vi "IMAQdxCam-Fast-TIFF.vi"() -> ()   [LabVIEW 2011]
uses:
  <vilib>/vision/driver/IMAQdx.llb/IMAQdx Acquisition Mode.ctl
  <vilib>/vision/driver/IMAQdx.llb/IMAQdx Buffer Number Mode.ctl
  tiff/TiffModules/AddTiffPage_U8_text_res.vi
  tiff/TiffModules/AddTiffPage_I16_text_res.vi
  <vilib>/vision/driver/NI_Vision_Acquisition_Software.lvlib
  C:/Program Files/National Instruments/LabVIEW 2011/resource/objmgr/imaqdx.rc
  C:/Program Files/National Instruments/LabVIEW 2011/resource/objmgr/IMAQImage.rc
panel:
  in  "Exposure":dbl(slide)=2689.598785575046 scale=100.0..100000.0
  in  "IMAQdx-Session":string="cam0"
  in  "expected images":u32=1
  out "msperframe":u32(graph)
  out "measured":i32
  out "saved":i32
  out "Buffer Number Out":u32
  out "IFDoffset":u32
  out "Image Type":i32(ring) items=["8 bits", "16 bits", "Float", "Complex", "RGB", "HSL"]
  out "measuredloop":i32
  in  "tiff-file":path=path "C:/temp/test1.tif"
  out "error out":errorcluster
  # "init the cam in MAX first!"
  # "wait for trigger will be enabled\nacquire as fast as possible to RAM (IMAQs)\nno diplay, \nsave afterwards"
  # "usually µs"
  # "0..."
  # "fast 8bit 3920x1848 1000us\ntested 7x50 (36,3fps 27ms)"
  # "I16 and U8 tested!\nwill overwrite! no append"
  # "init an test the cam with NiMax first! Find Session name\ngo gain etc with other"
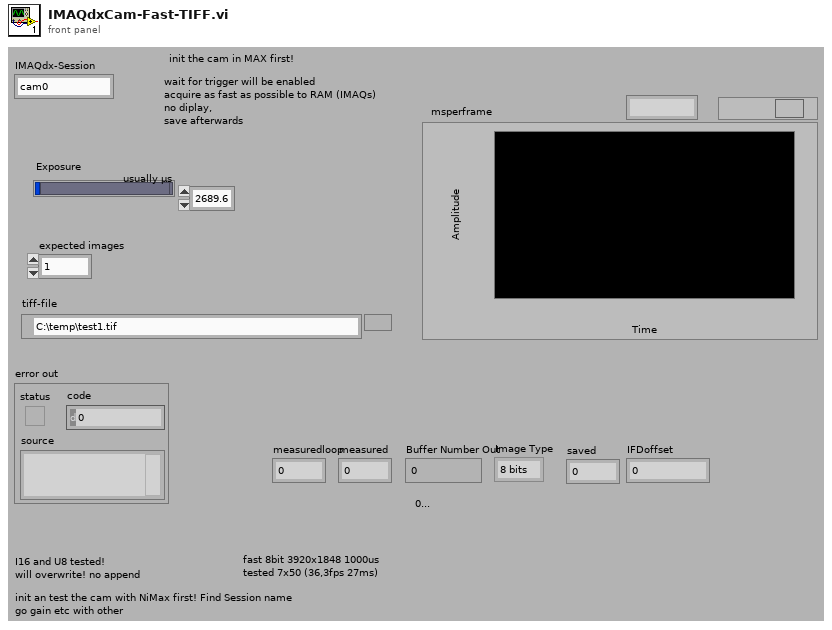
[diagram p1: front panel]
types:
  T1 = typedef "NI_Vision_Acquisition_Software.lvlib/IMAQdx Acquisition Mode.ctl" = enum32{"One Shot", "Continuous"}
  T2 = typedef "IMAQdx.ctl" = refnum<k21>
  T3 = typedef "Image Type" = u32
  T4 = typedef "IMAQ Image.ctl" = refnum<image>
  T5 = typedef "NI_Vision_Acquisition_Software.lvlib/IMAQdx Buffer Number Mode.ctl" = enum32{"Next", "Last", "Buffer Number"}
  T6 = cluster{"Tiff refnum":refnum<file>, "Byte-Reihenfolge (0:Big-Endian, 2:LSB)":enum16{"big-endian, network order", "native, host order", "little-endian"}}
  T7 = cluster{"Xpixelsize[µm]":sgl, "Ypixelsize[µm]":sgl}
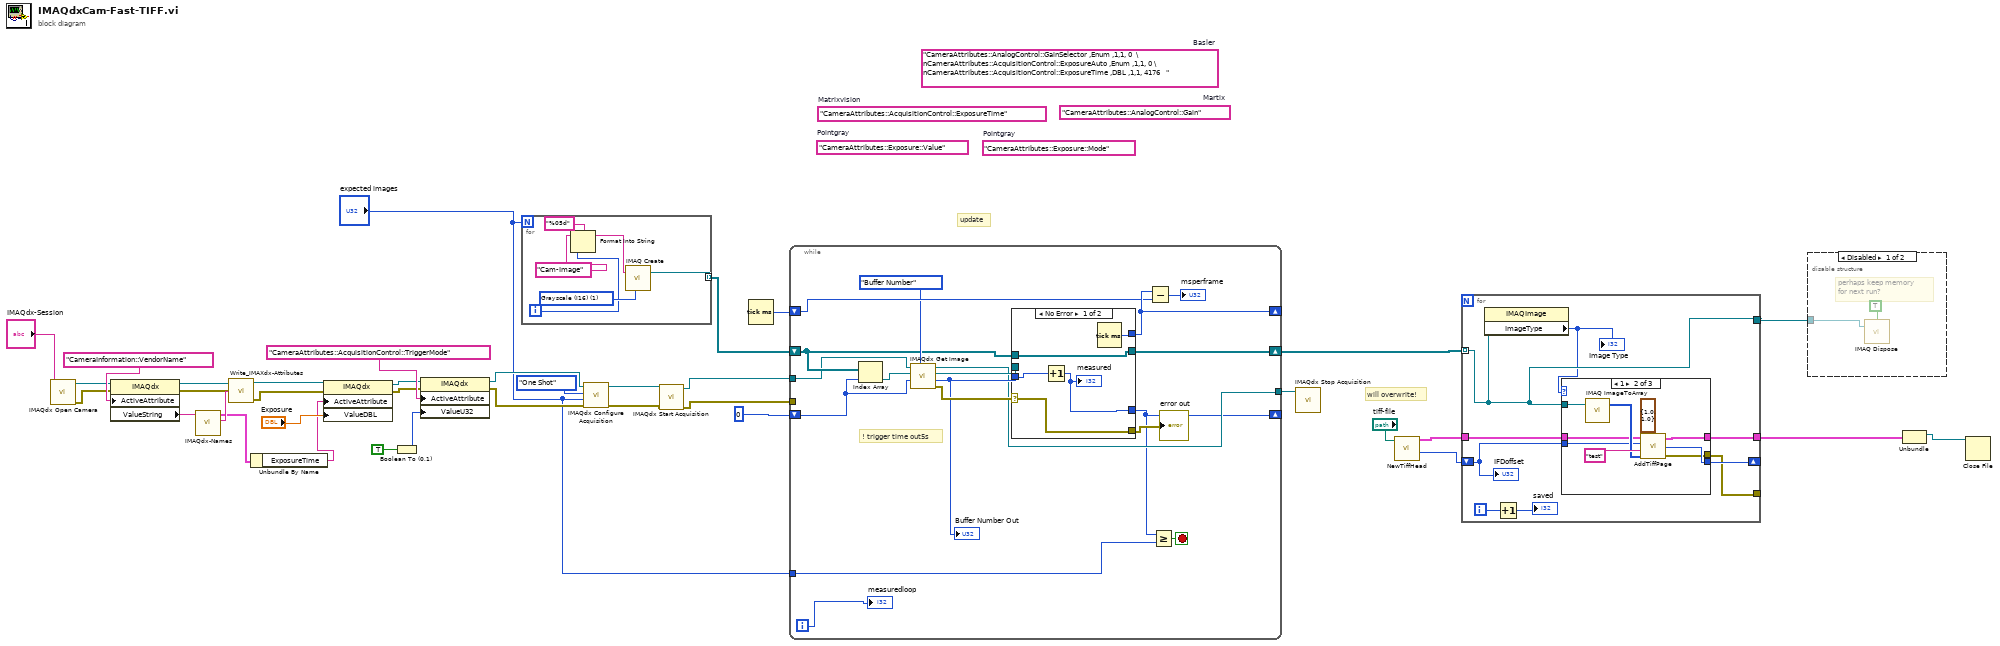
[diagram p0: block diagram]
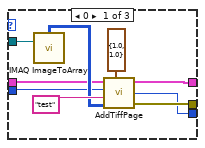
[diagram p3: hidden frame]
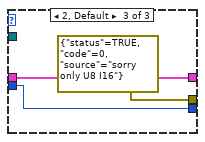
[diagram p4: hidden frame]
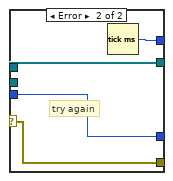
[diagram p5: hidden frame]
diagram:
  (unwired) "CameraAttributes::AnalogControl::Gain"  # Martix
  (unwired) "CameraAttributes::AnalogControl::GainSelector ,Enum ,1,1, 0  \nCameraAttributes::AcquisitionControl::ExposureAuto ,Enum ,1,1, 0 \nCameraAttributes::AcquisitionControl::ExposureTime ,DBL ,1,1, 4176   "  # Basler
  (unwired) "CameraAttributes::Exposure::Mode"  # Pointgray
  (unwired) "CameraAttributes::Exposure::Value"  # Pointgray
  (unwired) "CameraAttributes::AcquisitionControl::ExposureTime"  # Matrixvision
  # "update"
  # "will overwrite!"
  n1 = call <vilib>:"IMAQdx Open Camera.vi"("Session In"="IMAQdx-Session") -> ("error out"=w17:errorcluster, "Session Out"=w20:T2)  [unwired: 2 in, 7 out]
  n2 = property class="IMAQdx"(reference=w20, error in=w17, "ActiveAttribute"="CameraInformation::VendorName") -> (reference out=w19:T2, error out=w18:errorcluster, "ValueString"=w26:string)
  n3 = call "IMAQdx-Names.vi"("exactCameraName"=w26) -> ("Defaults"=w25:string, "shortcuts"=w16:cluster{"ExposureTime":string, "Gain":string})  [unwired: 8 in, 1 out]
  n4 = call "Write_IMAXdx-Attributes.vi"("error in"=w18, "IMAQdx-Defaults"=w25, "Session In"=w19) -> ("error out"=w15:errorcluster, "Session Out"=w9:T2)  [unwired: 1 in]
  n5 = Unbundle By Name(w16) -> ("ExposureTime"=w14:string)
  n6 = property class="IMAQdx"(reference=w9, error in=w15, "ActiveAttribute"=w14, "ValueDBL"="Exposure") -> (reference out=w13:T2, error out=w12:errorcluster)
  n7 = Boolean To (0,1)(Boolean=TRUE) -> (0, 1=w32:i16)
  n8 = property class="IMAQdx"(reference=w13, error in=w12, "ActiveAttribute"="CameraAttributes::AcquisitionControl::TriggerMode", "ValueU32"=w32) -> (reference out=w11:T2, error out=w10:errorcluster)
  n9 = for {
    N: "expected images" -> [_]
    tunnel: [w42] -> w36 mode=indexing
    i -> [w41]
    w43 = T3 1 items=["Grayscale (U8)", "Grayscale (I16)", "Grayscale (SGL)", "Complex (CSG)", "RGB (U32)", "HSL (U32)", "RGB (U64)", "Grayscale (U16)"] ("Image Type")
    n10 = Format Into String(format string="%05d", initial string="Cam-Image" ("Image Name"), w41) -> (resulting string=w39:string)  [unwired: 1 in, 1 out]
    n11 = call "IMAQ Create"("Image Name"=w39, "Image Type"=w43) -> ("New Image"=w42:T4)  [unwired: 2 in, 2 out]
  }
  n12 = call <vilib>:"IMAQdx Configure Acquisition.vi"("error in"=w10, "Number of Buffers"="expected images", "Continuous?"=IMAQdx_Acquisition_Mode."One Shot", "Session In"=w11) -> ("error out"=w8:errorcluster, "Session Out"=w6:T2)  [unwired: 6 in]
  n13 = call <vilib>:"IMAQdx Start Acquisition.vi"("error in"=w8, "Session In"=w6) -> ("error out"=w7:errorcluster, "Session Out"=w5:T2)  [unwired: 8 in]
  n14 = Tick Count (ms)() -> (millisecond timer value=w4:u32)
  n15 = while {
    tunnel: w5 -> [w50]
    shift-right: [w60] -> w22
    shift-left: w36 -> [w55]
    shift-right: [w59] -> _
    shift-left: w4 -> [w58]
    shift-right: [w44] -> _
    shift-left: u32 0 ("Buffer Number Out") -> [w45]
    tunnel: w7 -> [_]
    tunnel: [w49] -> w3
    tunnel: "expected images" -> [w48]
    i -> [w51]
    stop <- w47 stop-if-true
    # "! trigger time out5s"
    n16 = Index Array(array=w55, index=w45) -> (element=w54:T4)
    n17 = call <vilib>:"IMAQdx Get Image.vi"("Buffer Number Mode (Next)"=IMAQdx_Buffer_Number_Mode."Buffer Number", "Buffer Number In"=w45, "Image In"=w54, "Session In"=w50) -> ("error out"=w53:errorcluster, "Buffer Number Out"=w52:u32, "Image Out"=w57:T4, "Session Out"=w49:T2)  [unwired: 4 in]
    "Buffer Number Out" <- w52
    n18 = case shown="No Error" w53 {
      selector: w53 -> [w62 w67]
      tunnel: w57 -> [_ _]
      tunnel: [w62 w67] -> w61
      tunnel: w55 -> [w63 w70]
      tunnel: [w63 w70] -> w60
      tunnel: [w66 w69] -> w59
      tunnel: w52 -> [w65 w68]
      tunnel: [w64 w68] -> w44
      frame No Error {
        n19 = Increment(x=w65) -> (x+1=w64:u32)
        "measured" <- w64
        n20 = Tick Count (ms)() -> (millisecond timer value=w66:u32)
      }
      frame Error {
        # "try again"
        n21 = Tick Count (ms)() -> (millisecond timer value=w69:u32)
      }
    }
    "error out" <- w61
    n22 = Subtract(x=w59, y=w58) -> (x-y=→"msperframe":u32)
    n23 = Greater Or Equal?(x=w44, y=w48) -> (x >= y?=w47:bool)
    "measuredloop" <- w51
  }
  n24 = call <vilib>:"IMAQdx Stop Acquisition.vi"("Session In"=w3) -> ()  [unwired: 1 in, 10 out]
  n25 = call "NewTiffHead.vi"("file path"="tiff-file") -> ("TIFF file"=w24:T6, "Place for first IFD (8,eof-position)"=w23:u32)  [unwired: 2 in, 2 out]
  n26 = for {
    tunnel: w24 -> [w79]
    shift-right: [w77] -> _
    shift-left: w23 -> [w78]
    tunnel: [w76] -> _
    tunnel: w22 -> [w72] mode=indexing
    tunnel: [w75] -> w21
    tunnel: [w72] -> w1
    i -> [w74]
    n27 = property class="IMAQImage"(reference=w72) -> ("ImageType"=w71:i32)  [unwired: 1 in, 2 out]
    "Image Type" <- w71
    n28 = Increment(x=w74) -> (x+1=→"saved":i32)
    n29 = case shown="1" w71 {
      tunnel: w79 -> [w85 w95 w100]
      tunnel: w78 -> [w84 w94 w99]
      tunnel: [w82 w93 w99] -> w77
      tunnel: [w83 w92 errorcluster {"status"=TRUE, "code"=0, "source"="sorry only U8 I16"} ("error out")] -> w76
      tunnel: [w81 w91 w100] -> w75
      tunnel: w72 -> [w87 w90 _]
      frame 0 {
        n30 = call "IMAQ ImageToArray"("Image"=w87) -> ("Image Pixels (U8)"=w86:u8[][])  [unwired: 3 in, 4 out]
        n31 = call-poly "AddTiffPage.vi"("TIFF file"=w85, "After last DIROffset"=w84, "Text"="test", "16-bit pixmap x, y"=w86, "Pixelsize [µm]"=T7 {"Xpixelsize[µm]"=1.0, "Ypixelsize[µm]"=1.0}) -> ("TIFF file out"=w81:T6, "AfterDIRoffset"=w82:u64, "error out"=w83:errorcluster)
      }
      frame 1 {
        n32 = call "IMAQ ImageToArray"("Image"=w90) -> ("Image Pixels (I16)"=w96:i16[][])  [unwired: 3 in, 4 out]
        n33 = call-poly "AddTiffPage.vi"("TIFF file"=w95, "After last DIROffset"=w94, "Text"="test", "16-bit pixmap x, y"=w96, "Pixelsize [µm]"=T7 {"Xpixelsize[µm]"=1.0, "Ypixelsize[µm]"=1.0}) -> ("TIFF file out"=w91:T6, "AfterDIRoffset"=w93:u64, "error out"=w92:errorcluster)
      }
      frame 2, Default {
      }
    }
    "IFDoffset" <- w78
  }
  n34 = disable-structure shown="Disabled" {
    disable-tunnel: w1 -> [w102 _]
    frame Disabled {
      # "perhaps keep memory\nfor next run?"
      n35 = call "IMAQ Dispose"("All Images? (No)"=TRUE, "Image"=w102) -> ()  [unwired: 4 in, 1 out]
    }
    frame Enabled {
    }
  }
  n36 = Unbundle(w21) -> ("Tiff refnum"=w29:refnum<file>)  [unwired: 1 out]
  n37 = Close File(refnum=w29) -> ()  [unwired: 1 in, 2 out]
